vi "Get Next Run.vi"(8 "error in (no error)":errorcluster, 11 "Schedule in":refnum<class "Schedule.lvclass">) -> (0 "error out":errorcluster, 2 "Run Instance":refnum<class "Run Instance.lvclass">, 3 "Schedule out":refnum<class "Schedule.lvclass">)   [LabVIEW 2020, in "Run Utilities.lvlib" / "Schedule.lvclass"]
doc: "Takes out next RUN from the schedule. If there are no more repetitions of the RUN, it is removed from the array. Otherwise, it decreases number of repetitions by one"
uses:
  Schedule.lvclass
  Run Instance/Run Instance.lvclass
  Cell/Schedule Cell.lvclass
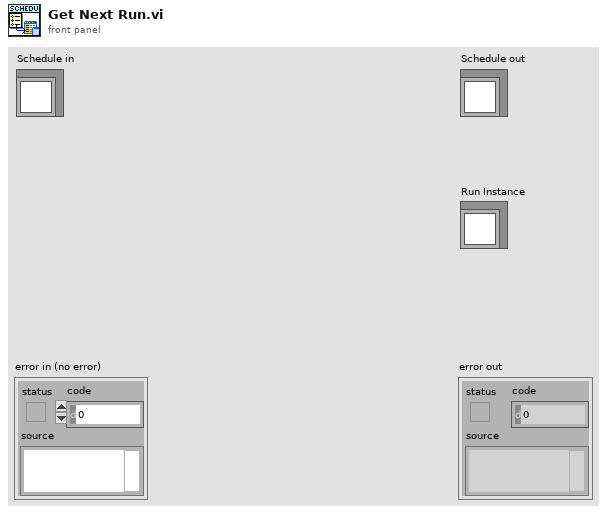
[diagram p1: front panel]
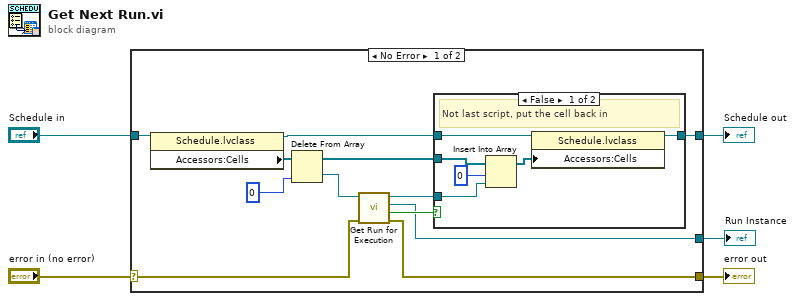
[diagram p0: block diagram]
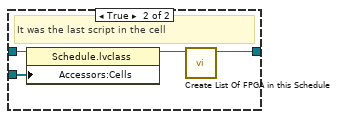
[diagram p2: hidden frame]
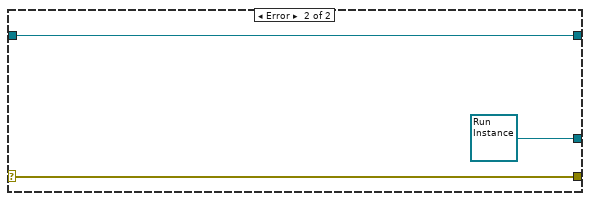
[diagram p3: hidden frame]
diagram:
  n1 = case shown="No Error" "error in (no error)" {
    selector: "error in (no error)" -> [w12 w30]
    tunnel: [w8 w30] -> w4
    tunnel: [w6 w29] -> w2
    tunnel: "Schedule in" -> [w17 w29]
    tunnel: [w9 refnum<class "Run Instance.lvclass"> refnum ("Run Instance")] -> w1
    frame No Error {
      n2 = property class="Schedule.lvclass"(reference=w17) -> (reference out=w7:refnum<class "Schedule.lvclass">, "Accessors:Cells"=w16:refnum<class "Schedule Cell.lvclass">[])  [unwired: 1 in, 1 out]
      n3 = Delete From Array(array=w16, index=0) -> (deleted portion=w13:refnum<class "Schedule Cell.lvclass">, array with subset deleted=w14:refnum<class "Schedule Cell.lvclass">[])  [unwired: 1 in]
      n4 = call-dynamic "Get Run for Execution.vi"("error in (no error)"=w12, "Schedule Cell in"=w13) -> ("error out"=w8:errorcluster, "Last Script"=w11:bool, "Run Instance"=w9:refnum<class "Run Instance.lvclass">, "Schedule Cell out"=w10:refnum<class "Schedule Cell.lvclass">)  [unwired: 6 in]
      n5 = case shown="False" w11 {
        tunnel: w14 -> [w22 w26]
        tunnel: w10 -> [w21 _]
        tunnel: w7 -> [w19 w27]
        tunnel: [w18 w25] -> w6
        frame False {
          # "Not last script, put the cell back in"
          n6 = Insert Into Array(array=w22, index=0, new element=w21) -> (w20:refnum<class "Schedule Cell.lvclass">[])
          n7 = property class="Schedule.lvclass"(reference=w19, "Accessors:Cells"=w20) -> (reference out=w18:refnum<class "Schedule.lvclass">)  [unwired: 1 in, 1 out]
        }
        frame True {
          # "It was the last script in the cell"
          n8 = property class="Schedule.lvclass"(reference=w27, "Accessors:Cells"=w26) -> (reference out=w24:refnum<class "Schedule.lvclass">)  [unwired: 1 in, 1 out]
          n9 = call-dynamic "Create List Of FPGA in this Schedule.vi"("Schedule in"=w24) -> ("Schedule out"=w25:refnum<class "Schedule.lvclass">)  [unwired: 9 in, 1 out]
        }
      }
    }
    frame Error {
    }
  }
  "error out" <- w4
  "Schedule out" <- w2
  "Run Instance" <- w1
